vi "Read Address.vi"(8 "error in":errorcluster, 11 "address ref in":refnum<k20>) -> (0 "error out":errorcluster, 2 "terminal":T1, 3 "address ref out":refnum<k20>)   [LabVIEW 2020, in "AIM MIL-STD 1553 Import.lvlib"]
uses:
  AIM MIL-STD 1553 Import.lvlib
  d1480715-b761-474b-8fe5-ec7c306e7985.vi
  e39d4d0c-c6d5-4d8d-a621-4ae47de02d87.vi
  Shared/Address.ctl
  Shared/Terminal Endpoint.ctl
  Constants.vi
  cef1b9ea-8129-4b98-8421-c923908517a8.vi
  68acfba6-3310-4a68-92ee-9cd7e900ed40.vi
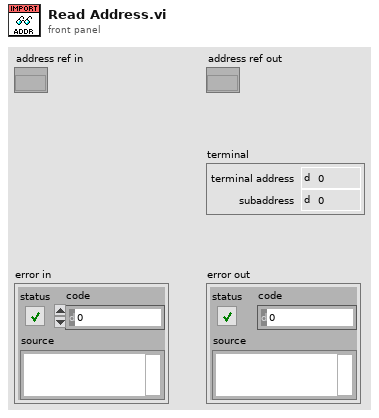
[diagram p1: front panel]
types:
  T1 = typedef "Terminal Endpoint.ctl" = cluster{"terminal address":T2, "subaddress":T2}
  T2 = typedef "Address.ctl" = u16
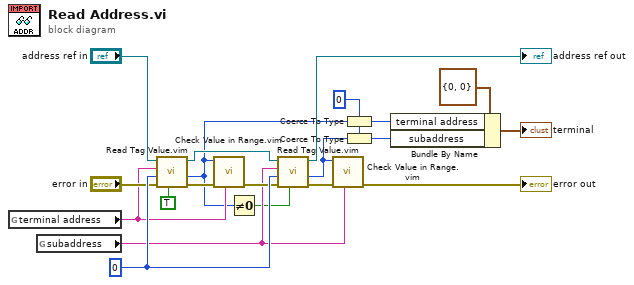
[diagram p0: block diagram]
diagram:
  w20 = u16 0 ("error code (0)")
  w17 = T2 0 ("subaddress")
  n1 = global read "Constants.vi" "terminal address"() -> (w4:string)
  n2 = global read "Constants.vi" "subaddress"() -> (w5:string)
  n3 = call "Read Tag Value.vim"("required (F)"=TRUE, "error in"="error in", "default"=w20, "tag name"=w4, "node in"="address ref in") -> ("error out"=w10:errorcluster, "value"=w2:u16, "node out"=w13:refnum<k20>)  [unwired: 4 in]
  n4 = call "Check Value in Range.vim"("element name"=w4, "error in"=w10, "value"=w2) -> ("error out"=w9:errorcluster)  [unwired: 8 in]
  n5 = Not Equal To 0?(x=w2) -> (x != 0?=w1:bool)
  n6 = call "Read Tag Value.vim"("required (F)"=w1, "error in"=w9, "default"=w20, "tag name"=w5, "node in"=w13) -> ("error out"=w8:errorcluster, "value"=w3:u16, "node out"=→"address ref out":refnum<k20>)  [unwired: 4 in]
  n7 = call "Check Value in Range.vim"("element name"=w5, "error in"=w8, "value"=w3) -> ("error out"=→"error out":errorcluster)  [unwired: 8 in]
  n8 = Coerce To Type(0:w2, 1:w17) -> (2:w15:T2)
  n9 = Coerce To Type(0:w3, 1:w17) -> (2:w16:T2)
  n10 = Bundle By Name(cluster=T1 {"terminal address"=0, "subaddress"=0} ("endpoint Rx"), "terminal address"=w15, "subaddress"=w16) -> (→"terminal":T1)
